vi "Case_Selector.vi"(11 "Array":bool[](array[boolean])) -> (3 "Case Numer":i32)   [LabVIEW 2014]
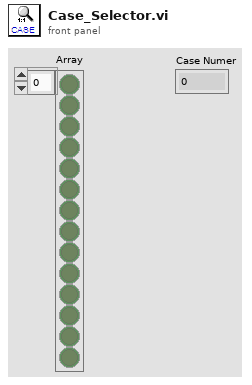
[diagram p1: front panel]
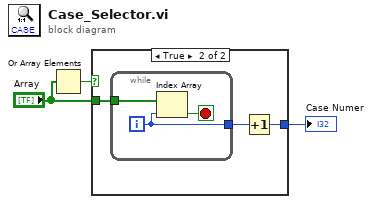
[diagram p0: block diagram]
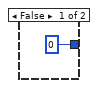
[diagram p2: hidden frame]
diagram:
  n1 = Or Array Elements(Boolean array="Array") -> (logical OR=w3:bool)
  n2 = case shown="True" w3 {
    tunnel: [0 w5] -> w2
    tunnel: "Array" -> [_ w7]
    frame False {
    }
    frame True {
      n3 = while {
        tunnel: w7 -> [w10]
        tunnel: [w8] -> w6
        i -> [w8]
        stop <- w9 stop-if-true
        n4 = Index Array(array=w10, index=w8) -> (element=w9:bool)
      }
      n5 = Increment(x=w6) -> (x+1=w5:i32)
    }
  }
  "Case Numer" <- w2
